vi "Coersion Dot.vi"() -> ()   [LabVIEW 2019]
panel:
  out "Numeric 2":i32
  in  "Numeric":i8
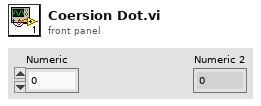
[diagram p1: front panel]
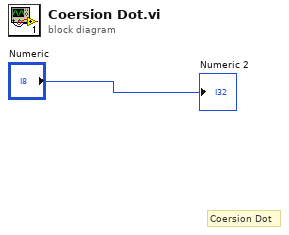
[diagram p0: block diagram]
diagram:
  # "Coersion Dot"
  "Numeric 2" <- "Numeric"
